vi "PicoScope2000aWrapSettings.vi"(4 "Device Info":T1, 9 "Enabled array":i16[](array[numeric]), 10 "Handle In":i16, 11 "error in (no error)":errorcluster) -> (2 "Handle Out":i16, 3 "error out":errorcluster)   [LabVIEW 2010]
uses:
  ps2000aWrap.dll
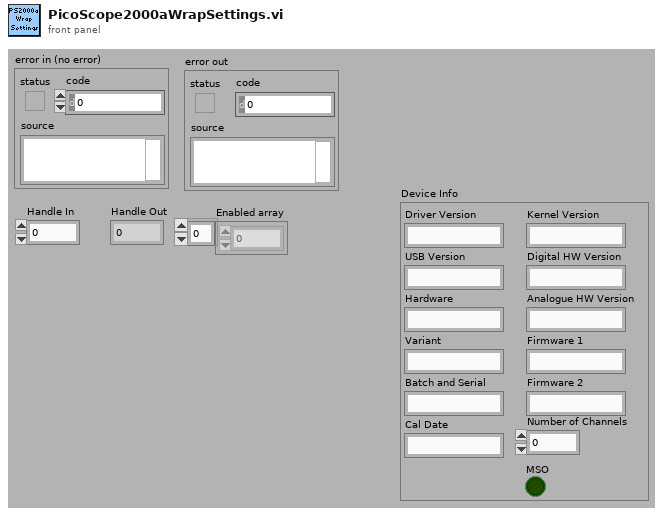
[diagram p1: front panel]
types:
  T1 = cluster{"Driver Version":string, "USB Version":string, "Hardware":string, "Variant":string, "Batch and Serial":string, "Cal Date":string, "Kernel Version":string, "Digital HW Version":string, "Analogue HW Version":string, "Firmware 1":string, "Firmware 2":string, "MSO":bool, "Number of Channels":i16}
  T2 = cluster{"status":bool, "code":u32, "source":string}
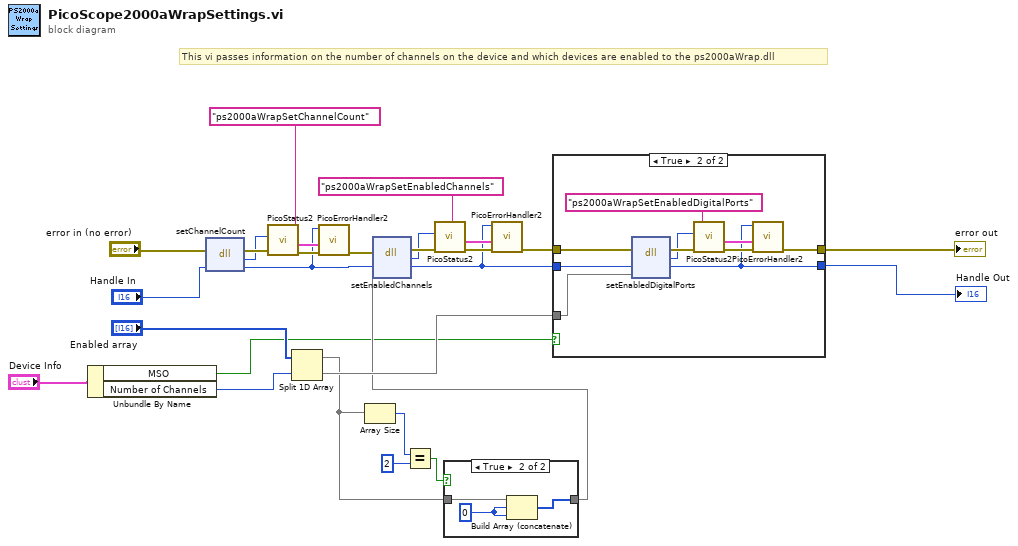
[diagram p0: block diagram]
diagram:
  # "This vi passes information on the number of channels on the device and which devices are enabled to the ps2000aWrap.dll"
  n1 = Unbundle By Name("Device Info") -> ("MSO"=w8:bool, "Number of Channels"=w11:i16)
  n2 = dll-call lib="ps2000aWrap.dll" fn="setChannelCount"(error in="error in (no error)", "handle"="Handle In") -> (error out=w24:errorcluster, "PICO_STATUS"=w23:u32, "handle"=w3:i16)  [unwired: 2 in, 1 out]
  n3 = call "PicoStatus2.vi"("PICO source"="ps2000aWrapSetChannelCount" ("source"), "Error in"=w24, "PICO STATUS"=w23) -> ("error out"=w5:errorcluster, "PICO_STATUS out"=w4:T2)  [unwired: 5 in]
  n4 = Split 1D Array(array="Enabled array", index=w11) -> (first subarray=w10:i16[], second subarray=w16:i16[])
  n5 = call "PicoErrorHandler2.vi"("error in (no error)"=w5, "PICO_STATUS in"=w4, "handle In"=w3) -> ("error out"=w2:errorcluster)  [unwired: 8 in]
  n6 = Array Size(array=w10) -> (size(s)=w13:i32)
  n7 = Equal?(x=w13, y=2) -> (x = y?=w14:bool)
  n8 = case shown="True" w14 {
    tunnel: w10 -> [w29 w32]
    tunnel: [w29 w30] -> w9
    frame False {
    }
    frame True {
      w31 = i16 0 ("y")
      n9 = Build Array (concatenate)(w32, w31, w31) -> (w30:i16[])
    }
  }
  n10 = dll-call lib="ps2000aWrap.dll" fn="setEnabledChannels"(error in=w2, "handle"=w3, "enabledChannels"=w9) -> (error out=w27:errorcluster, "PICO_STATUS"=w26:u32, "handle"=w6:i16)  [unwired: 3 in, 1 out]
  n11 = call "PicoStatus2.vi"("PICO source"="ps2000aWrapSetEnabledChannels" ("source"), "Error in"=w27, "PICO STATUS"=w26) -> ("error out"=w28:errorcluster, "PICO_STATUS out"=w7:T2)  [unwired: 5 in]
  n12 = call "PicoErrorHandler2.vi"("error in (no error)"=w28, "PICO_STATUS in"=w7, "handle In"=w6) -> ("error out"=w17:errorcluster)  [unwired: 8 in]
  n13 = case shown="True" w8 {
    tunnel: w6 -> [w34 w41]
    tunnel: w17 -> [w33 w40]
    tunnel: [w33 w37] -> w1
    tunnel: [w34 w35] -> w18
    tunnel: w16 -> [_ w39]
    frame False {
    }
    frame True {
      n14 = dll-call lib="ps2000aWrap.dll" fn="setEnabledDigitalPorts"(error in=w40, "handle"=w41, "enabledDigitalPorts"=w39) -> (error out=w44:errorcluster, "PICO_STATUS"=w43:u32, "handle"=w35:i16)  [unwired: 3 in, 1 out]
      n15 = call "PicoStatus2.vi"("PICO source"="ps2000aWrapSetEnabledDigitalPorts" ("source"), "Error in"=w44, "PICO STATUS"=w43) -> ("error out"=w38:errorcluster, "PICO_STATUS out"=w36:T2)  [unwired: 5 in]
      n16 = call "PicoErrorHandler2.vi"("error in (no error)"=w38, "PICO_STATUS in"=w36, "handle In"=w35) -> ("error out"=w37:errorcluster)  [unwired: 8 in]
    }
  }
  "Handle Out" <- w18
  "error out" <- w1
